vi "Instrument Update for Spartan 5.0.vi"(8 "error in (no error)":errorcluster, 10 "Old Instrument Record":T1) -> (0 "error out":errorcluster, 2 "New Instrument Record":T1)   [LabVIEW 2011]
uses:
  Instrument Record.ctl
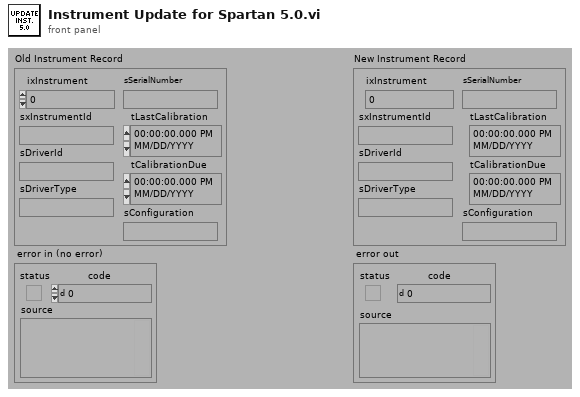
[diagram p1: front panel]
types:
  T1 = typedef "Instrument Record.ctl" = cluster{"ixInstrument":i32, "sxInstrumentId":string, "sDriverId":string, "sDriverType":string, "sSerialNumber":string, "tLastCalibration":timestamp, "tCalibrationDue":timestamp, "sConfiguration":string}
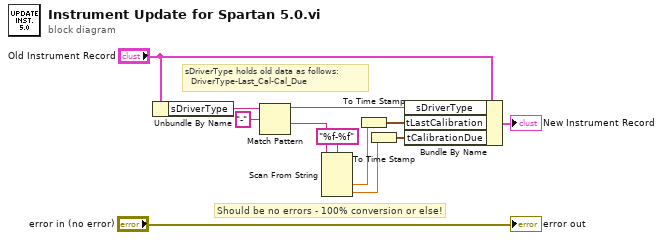
[diagram p0: block diagram]
diagram:
  # "sDriverType holds old data as follows:\n  DriverType-Last_Cal-Cal_Due"
  # "Should be no errors - 100% conversion or else!"
  n1 = Unbundle By Name("Old Instrument Record") -> ("sDriverType"=w7:string)
  n2 = Match Pattern(string=w7, regular expression="-") -> (before substring=w5:string, after substring=w8:string)  [unwired: 3 out]
  n3 = Scan From String(format string="%f-%f", input string=w8) -> (output 1=w4:dbl, output 2=w2:dbl)  [unwired: 2 in, 5 out]
  n4 = To Time Stamp(1:w4) -> (0:w3:timestamp)
  n5 = To Time Stamp(1:w2) -> (0:w1:timestamp)
  n6 = Bundle By Name(cluster="Old Instrument Record", "sDriverType"=w5, "tLastCalibration"=w3, "tCalibrationDue"=w1) -> (→"New Instrument Record":T1)
  "error out" <- "error in (no error)"
